vi "change-file-extension-name-subvi.vi"(2 "New Extension (no period)":string="html", 3 "Path String In":string) -> (0 "New Path String Out":string, 1 "New Path Out":path)   [LabVIEW 2014]
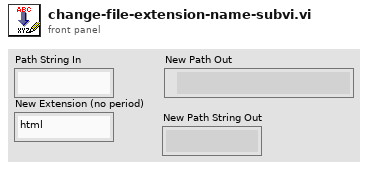
[diagram p1: front panel]
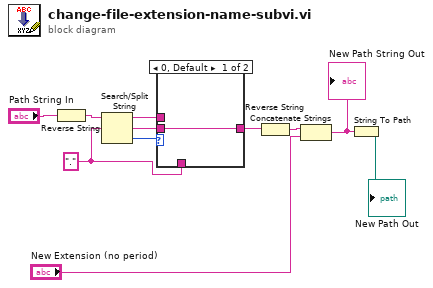
[diagram p0: block diagram]
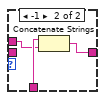
[diagram p2: hidden frame]
diagram:
  w2 = "." ("search string/char (-)")
  n1 = Reverse String(1:"Path String In") -> (0:w7:string)
  n2 = Search/Split String(string=w7, search string/char (-)=w2) -> (substring before match=w1:string, match + rest of string=w4:string, offset of match=w5:i32)  [unwired: 1 out]
  n3 = case shown="0, Default" w5 {
    tunnel: w4 -> [w12 _]
    tunnel: [w12 w13] -> w3
    tunnel: w2 -> [_ w15]
    tunnel: w1 -> [_ w14]
    frame 0, Default {
    }
    frame -1 {
      n4 = Concatenate Strings(w15, w14) -> (w13:string)
    }
  }
  n5 = Reverse String(1:w3) -> (0:w8:string)
  n6 = Concatenate Strings(w8, "New Extension (no period)") -> (w10:string)
  "New Path String Out" <- w10
  n7 = String To Path(string=w10) -> (path=→"New Path Out":path)
